vi "Example.vi"(8 "Error In":errorcluster) -> (0 "Error Out":errorcluster)   [LabVIEW 2017, in "TwinCAT ADS.lvlib"]
uses:
  TwinCAT ADS.lvlib
  TypeDefs/AMS.ctl
  1c5535b3-2415-44f7-bff6-c9bddd6bc487.vi
  High Level/PLC/Helpers/Variant to Byte Array.vi
  High Level/ADS Command/Read Write.vi
  ADS Errors.vi
  High Level/PLC/Helpers/Reorder Byte Array.vi
  High Level/PLC/PLC.lvlib
panel:
  in  "OK Button":bool
  in  "Stop Button":bool
  in  "Numeric Control":u16[][](array[numeric])
  in  "AMS":T1={"Target Net ID"="10.0.3.5.1.1", "Target Port"=10000, "Source Net ID"="192.168.56.1.1.1", "Source Port"=10000}
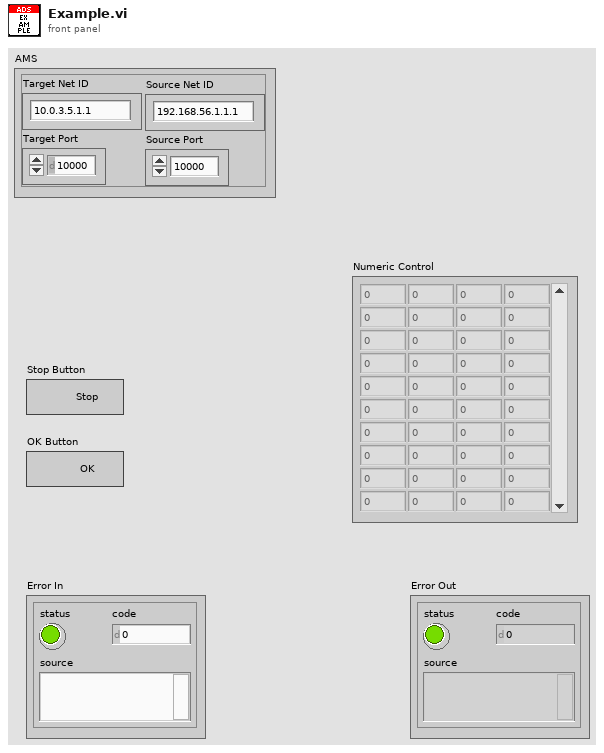
[diagram p1: front panel]
types:
  T1 = typedef "TwinCAT ADS.lvlib/AMS.ctl" = cluster{"Target Net ID":string, "Target Port":u16, "Source Net ID":string, "Source Port":u16}
  T2 = typedef "TwinCAT ADS.lvlib/AMS Connection.ctl" = cluster{"AMS":T1, "Timeout":i32, "TCP Connection Ref":refnum<k5>}
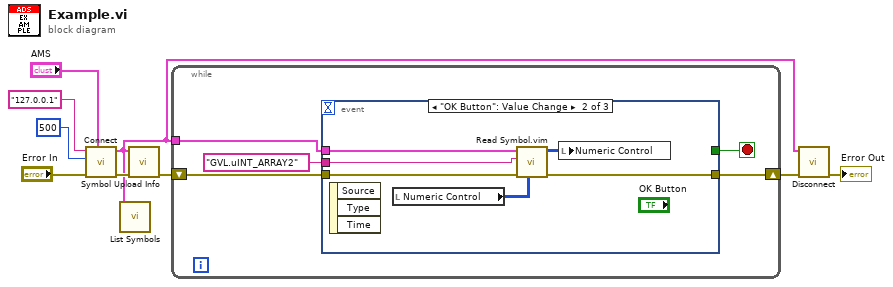
[diagram p0: block diagram]
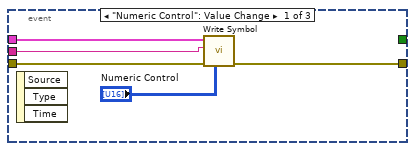
[diagram p2: hidden frame]
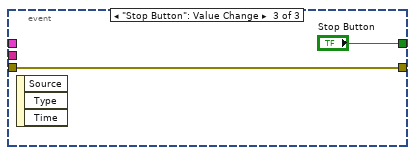
[diagram p3: hidden frame]
diagram:
  n1 = call "Connect.vi"("AMS"="AMS", "Error In"="Error In", "Timeout"=500, "Router"="127.0.0.1") -> ("Error Out"=w2:errorcluster, "AMS Connection"=w1:T2)  [unwired: 4 in, 2 out]
  n2 = call "List Symbols.vi"("AMS Connection In"=w1) -> ()  [unwired: 9 in, 2 out]
  n3 = call "Symbol Upload Info.vi"("Error In"=w2, "AMS Connection In"=w1) -> ("Error Out"=w4:errorcluster)  [unwired: 7 in, 2 out]
  n4 = while {
    tunnel: w1 -> [w14]
    shift-right: [w12] -> w3
    shift-left: w4 -> [w13]
    stop <- w11 stop-if-true
    n5 = event shown="[1] \"OK Button\": Value Change" {
      selector: _ -> [_ _ _]
      dyn-events: _ -> [_ _ _]
      timeout: _ -> [_ _ _]
      tunnel: w13 -> [w19 w21 w26]
      tunnel: w14 -> [w18 w25 _]
      tunnel: [w17 w20 w26] -> w12
      tunnel: [_ _ "Stop Button"] -> w11
      tunnel: "GVL.uINT_ARRAY2" ("Symbol Name") -> [w15 w24 _]
      event "Numeric Control": Value Change {
        n6 = event-data() -> ()  [unwired: 1 in, 3 out]
        n7 = call "Write Symbol.vi"("Data"="Numeric Control", "Error In"=w19, "Symbol Name"=w15, "AMS Connection"=w18) -> ("Error Out"=w17:errorcluster)  [unwired: 7 in]
      }
      event "OK Button": Value Change {
        n8 = event-data() -> ()  [unwired: 1 in, 3 out]
        n9 = local read "Numeric Control"() -> (w22:u16[][])
        n10 = call "Read Symbol.vim"("Data Type"=w22, "Error In"=w21, "Symbol Name"=w24, "AMS Connection In"=w25) -> ("Error Out"=w20:errorcluster, "Data"=w23:u16[][])  [unwired: 6 in]
        n11 = local write "Numeric Control"(w23) -> ()
      }
      event "Stop Button": Value Change {
        n12 = event-data() -> ()  [unwired: 1 in, 3 out]
      }
    }
  }
  n13 = call "Disconnect.vi"("Error In"=w3, "AMS Connection"=w1) -> ("Error Out"=→"Error Out":errorcluster)  [unwired: 9 in]
